vi "Read max value.vi"(8 "error in (no error)":errorcluster, 11 "Motor in":refnum<class "Motor.lvclass">) -> (0 "error out":errorcluster, 1 "max value":string, 2 "position":string, 3 "Motor out":refnum<class "Motor.lvclass">)   [LabVIEW 2018, in "Motor.lvclass"]
uses:
  Motor.lvclass
  Motor.lvclass/Motor.ctl
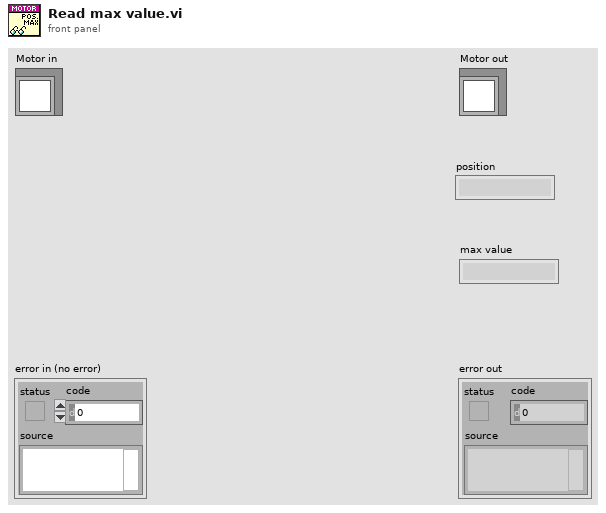
[diagram p1: front panel]
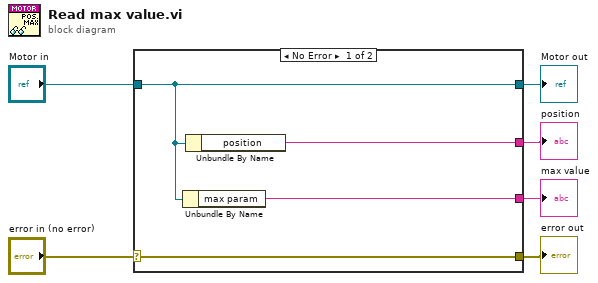
[diagram p0: block diagram]
diagram:
  n1 = case shown="No Error" "error in (no error)" {
    selector: "error in (no error)" -> [w10 w11]
    tunnel: [w10 w11] -> w5
    tunnel: [w8 w12] -> w3
    tunnel: "Motor in" -> [w8 w12]
    tunnel: [w9 _] -> w2
    tunnel: [w7 _] -> w1
    frame No Error {
      n2 = Unbundle By Name(w8) -> ("max param"=w9:string)
      n3 = Unbundle By Name(w8) -> ("position"=w7:string)
    }
    frame Error {
    }
  }
  "error out" <- w5
  "Motor out" <- w3
  "max value" <- w2
  "position" <- w1
